vi "Set Strings from Ref.vi"(8 "error in (no error)":errorcluster, 9 "Language Index (0)":i32, 10 "GObj Refnum":refnum<vi>, 11 "ArrayConstant in":refnum<class "ArrayConstant.lvclass">) -> (0 "error out":errorcluster, 3 "ArrayConstant out":refnum<class "ArrayConstant.lvclass">)   [LabVIEW 2013, in "SET Project Data.lvlib" / "ArrayConstant.lvclass"]
uses:
  ArrayConstant.lvclass
  GObject/GObject.lvclass
  SET Project Data.lvlib
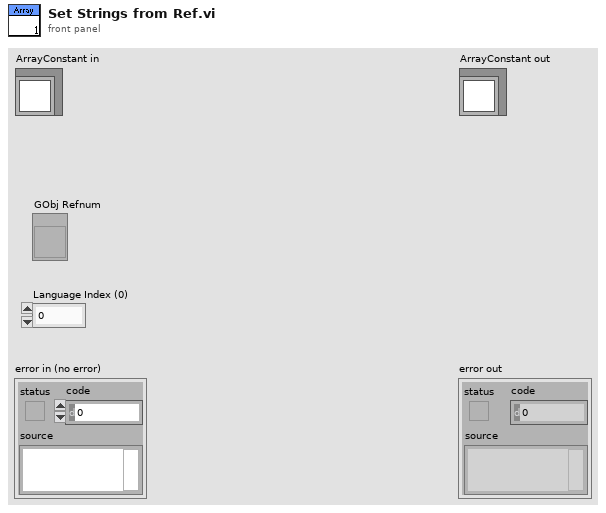
[diagram p1: front panel]
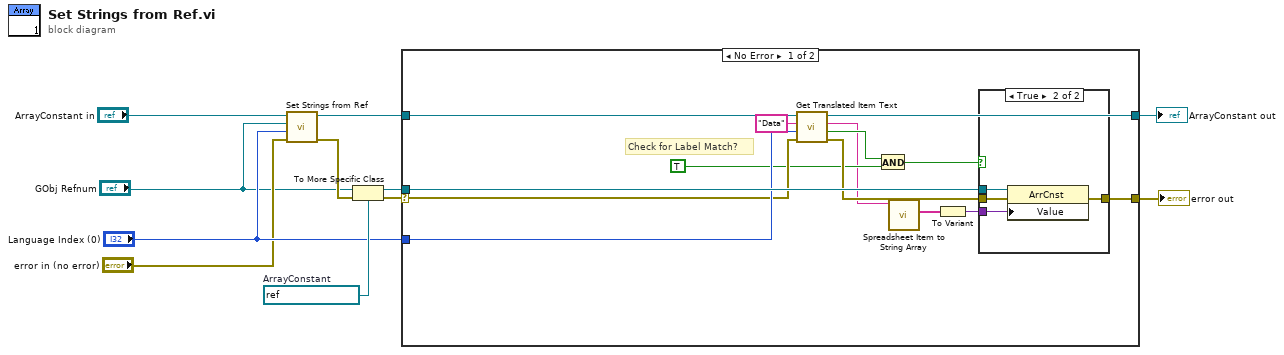
[diagram p0: block diagram]
diagram:
  w8 = refnum<vi> refnum  # ArrayConstant
  n1 = call-parent "Set Strings from Ref.vi"("error in (no error)"="error in (no error)", "Language Index (0)"="Language Index (0)", "GObj Refnum"="GObj Refnum", "GObject in"="ArrayConstant in") -> ("error out"=w11:errorcluster, "GObject out"=w7:refnum<class "ArrayConstant.lvclass">)  [unwired: 6 in]
  n2 = To More Specific Class(target class=w8, reference="GObj Refnum", error in=w11) -> (specific class reference=w9:refnum<vi>, error out=w10:errorcluster)
  n3 = case shown="No Error" w10 {
    selector: w10 -> [w21 w31]
    tunnel: w9 -> [w25 _]
    tunnel: w7 -> [w24 w32]
    tunnel: [w22 w32] -> w1
    tunnel: "Language Index (0)" -> [w23 _]
    tunnel: [w20 w31] -> w2
    frame No Error {
      # "Check for Label Match?"
      n4 = call "Get Translated Item Text.vi"("error in (no error)"=w21, "LangIndex (0)"=w23, "ItemName"="Data", "GObject in"=w24) -> ("error out"=w18:errorcluster, "Found?"=w16:bool, "Translated Text (ASCII)"=w14:string, "GObject out"=w22:refnum<class "ArrayConstant.lvclass">)  [unwired: 4 in]
      n5 = And(x=w16, y=TRUE) -> (x .and. y?=w15:bool)
      n6 = call "Spreadsheet Item to String Array.vi"("Spreadsheet Item (ASCII)"=w14) -> ("Strings [] (ASCII)"=w13:string[])  [unwired: 10 in]
      n7 = To Variant(anything=w13) -> (Variant=w12:variant)
      n8 = case shown="True" w15 {
        tunnel: w25 -> [_ w30]
        tunnel: w12 -> [_ w29]
        tunnel: w18 -> [w26 w28]
        tunnel: [w26 w27] -> w20
        frame False {
        }
        frame True {
          n9 = property class="ArrCnst"(reference=w30, error in=w28, "Value"=w29) -> (error out=w27:errorcluster)  [unwired: 1 out]
        }
      }
    }
    frame Error {
    }
  }
  "error out" <- w2
  "ArrayConstant out" <- w1
